vi "WaitForEdge_Single.vi"() -> ()   [LabVIEW 2014]
doc: "This example VI demonstrates the use of GPIO interrupts to wait for an edge event on a single input. \n\nTo use this VI simply wire an appropriate LED between a GPIO channel and Ground. Supply the pin number (default = GPIO 24) to the Output channel control. Likewise wire a simple button to a different GPIO channel and supply that pin number to the Input channel control.\n\nBroadcom numbering for the GPIO pins is assumed by this VI.\n\nAfter wiring the circuit, deploy the VI to the Raspberry Pi and run it. When you push and/or release the button depending on the Edge setting, an event will be triggered and the output channel will be toggled. Multiple toggles with a single press are most likely the result of switch bouncing."
uses:
  controls/IO_Direction.ctl
panel:
  out "error out":errorcluster
  out "Value":bool
  in  "Stop":bool
  in  "Edge":enum16{"Rising", "Falling", "Both"}(ring)
  in  "Output channel":i32=24
  in  "Input channel":i32=25 caption="Output channel"
  # "Wire Button to GPIO Input Channel\nWire LED to Output Channel\n\nEdge detection toggles LED"
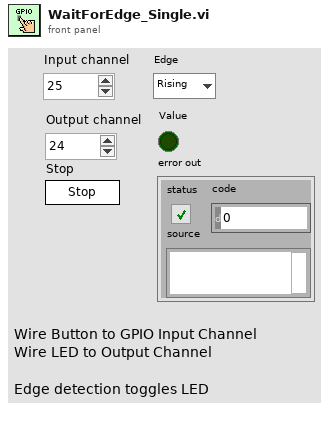
[diagram p1: front panel]
types:
  T1 = typedef "IO_Direction.ctl" = enum16{"Input", "Output"}
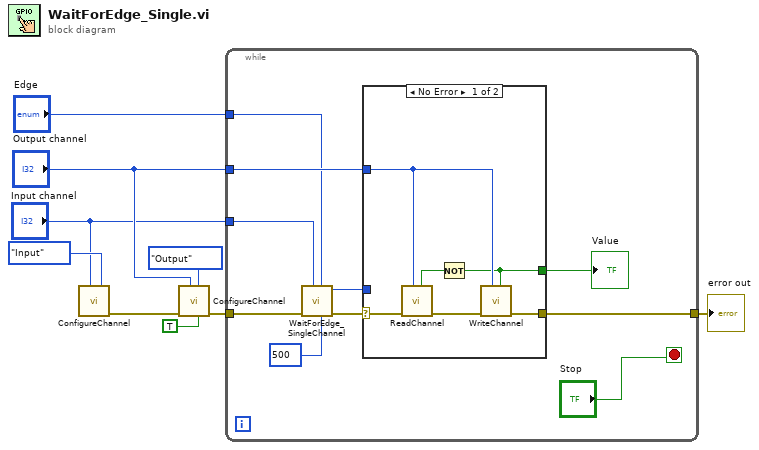
[diagram p0: block diagram]
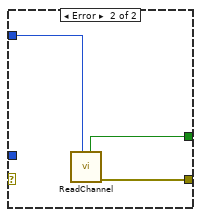
[diagram p2: hidden frame]
diagram:
  n1 = call "ConfigureChannel.vi"("Direction"=IO_Direction."Input", "Channel"="Input channel") -> ("error out"=w3:errorcluster)  [unwired: 9 in]
  n2 = call "ConfigureChannel.vi"("Initial value"=TRUE, "Direction"=IO_Direction."Output", "Channel"="Output channel", "error in"=w3) -> ("error out"=w7:errorcluster)  [unwired: 7 in]
  n3 = while {
    tunnel: w7 -> [w12]
    tunnel: "Input channel" -> [w15]
    tunnel: "Output channel" -> [w19]
    tunnel: "Edge" -> [w14]
    tunnel: [w17] -> w4
    stop <- "Stop" stop-if-true
    n4 = call "WaitForEdge_SingleChannel.vi"("Timeout (msec)"=500, "Edge"=w14, "Channel"=w15, "error in"=w12) -> ("error out"=w11:errorcluster, "Channel out"=w10:i32)  [unwired: 6 in]
    n5 = case shown="No Error" w11 {
      selector: w11 -> [w25 _]
      tunnel: w10 -> [_ _]
      tunnel: w19 -> [w21 w26]
      tunnel: [w23 w28] -> w17
      tunnel: [w20 w27] -> w18
      frame No Error {
        n6 = call "ReadChannel.vi"("Channel"=w21, "error in"=w25) -> ("error out"=w24:errorcluster, "Value"=w22:bool)  [unwired: 6 in]
        n7 = Not(x=w22) -> (.not. x?=w20:bool)
        n8 = call "WriteChannel.vi"("Value"=w20, "Channel"=w21, "error in"=w24) -> ("error out"=w23:errorcluster)  [unwired: 6 in]
      }
      frame Error {
        n9 = call "ReadChannel.vi"("Channel"=w26) -> ("error out"=w28:errorcluster, "Value"=w27:bool)  [unwired: 7 in]
      }
    }
    "Value" <- w18
  }
  "error out" <- w4
